vi "Wizard.vi"() -> ()   [LabVIEW 2014]
uses:
  TypeDef and Controls/QWizardMessage.ctl
  <vilib>/Utility/miscctls.llb/LVRowAndColumnUnsignedTypeDef.ctl
  Wizard Global Variable.vi
  <vilib>/Platform/browser.llb/Open URL in Default Browser (path).vi
  <vilib>/addons/_office/excel.llb/Excel Easy Table (str).vi
  <vilib>/Utility/NIReport.llb/NI_report.lvclass
  <vilib>/lvdsc/NI_DSC.lvlib
  <vilib>/addons/_office/NI_ReportGenerationToolkit.lvlib
panel:
  in  "Previous":bool
  in  "Cancel":bool
  in  "Next":bool
  in  "Tab Control":T1(tab)
  in  "Step 0 Selector":enum32{"Create", "Manage"}(radio) caption="Select an option to proceed"
  in  "what is database?":bool
  in  "Step 1 Database":enum32{"Database Ready", "Make Database"}(radio) caption="Select an option to proceed"
  out "S1 database def":string
  in  "S2 Library Name":string caption="Library Name"
  in  "S2 Database Location":path caption="Database Location"
  in  "S2 bool Library Name":enum32{"Libname:app", "Libname:user"}(radio) caption="Select an option to proceed"
  out "TextPage3":string
  in  "Bind":bool
  out "Processing 2":string
  out "S3 Status":string caption="Status"
  in  "S3 Open File Location":bool
  out "Processing":string
  in  "S4 Server IP":string="localhost" caption="Server Name/IP"
  in  "S4 Deployed Processes":i32[](listbox) caption="Deployed Processes"
  in  "S4 Remove Process":bool
  in  "S4 Get Process":bool
  in  "S4 Initialize":bool
  in  "S4 Deploy":bool
  in  "S4 SV Lib Path":path caption="Shared Variable Library Location"
  out "S5 Status":string caption="Status"
  in  "Redo":bool
  in  "Import":bool
  in  "Created Database":i32[](listbox) caption="Variables (in selected process)"
  in  "Variables":i32[](listbox) caption="Variables (in selected process)"
  in  "Deployed Pros. AP2":i32(listbox) caption="Deployed Processes"
  in  "Database Loc AP2":path caption="Database Location"
  in  "Database Name AP2":string caption="Database Name"
  # "SV Creation Wizard"
  # "This wizard assists you to create, deploy, and initialize shared variables."
  # "You have selected to create shared variables. You need to have a database."
  # "This application creates a LabVIEW library (*.lvlib) which contains shared variables. \nWhat shall be the name of the library?"
  # "The process to create shared varibles started ..."
  # "You can deploy and initialize the library.\n\nInitialization set booleans with False, strings with empty string, scalars with 0 of the same type, \n1D/2D arrays with 1D/2D arrays of size 1 with 0 or empty strings."
  # "Select a location  and a name to save the database."
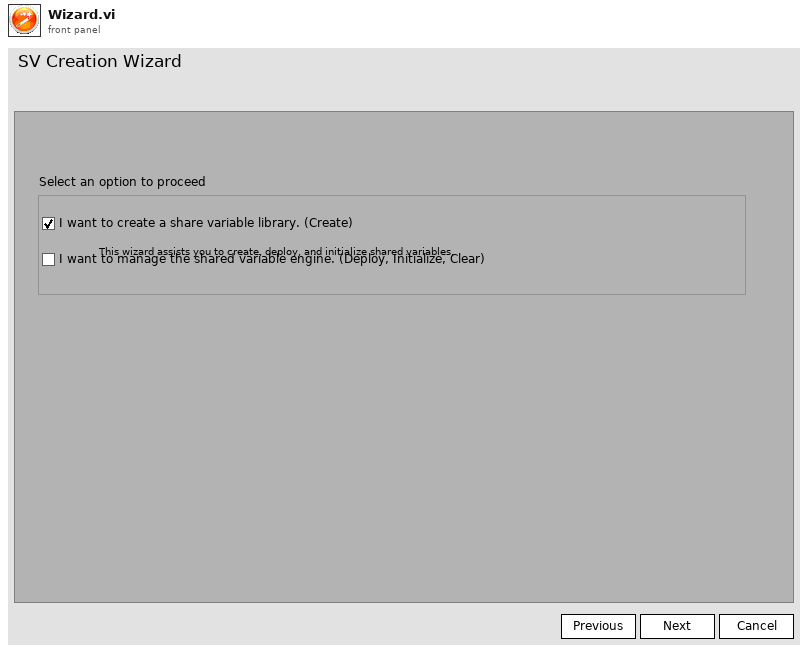
[diagram p1: front panel]
types:
  T1 = enum32{"Page 1", "Page 2", "Page 3", "Page 4", "Page 5", "Page 6", "Page 7"}
  T2 = cluster{"Number of Variables":i32, "Variable/Parent Name array":string[][], "URL array":string[], "Type array":string[]}
  T3 = typedef "QWizardMessage.ctl" = cluster{"State":enum16{"Initialize 0", "Initialize 1", "Initialize 2", "Initialize 3", "Initialize 4", "Back", "Next", "Check Database", "Get Lib Name", "Get Lib Folder", "Get Database", "Check Lib Availability", "Create SV Lib", "Check Binding", "Bind", "Get Processes", "Deploy", "Remove Process", "Clear Engine", "Initialize Process", "Get Process AP2", "Update Var AP2", "Import", "Redo", "Save Database", "Exit"}, "Data":variant}
  T4 = cluster{"Tab Pages Ref":refnum<vi>[], "Lib Name":string, "Lib Path":path, "Data":string[][], "Lib Full Path":path, "Deployed Processes":string[], "SV Info for Process":cluster{"Number of Variables":i32, "Variable/Parent Name array":string[][], "URL array":string[], "Type array":string[]}}
  T5 = typedef "LVRowAndColumnUnsignedTypeDef.ctl" = cluster{"Row":u32, "Column":u32}
  T6 = enum16{"Standard Report", "HTML", "Word", "Excel"}
  T7 = enum16{"maximized", "minimized", "normal", "no change"}
  T8 = enum16{"Initialize 0", "Initialize 1", "Initialize 2", "Initialize 3", "Initialize 4", "Back", "Next", "Check Database", "Get Lib Name", "Get Lib Folder", "Get Database", "Check Lib Availability", "Create SV Lib", "Check Binding", "Bind", "Get Processes", "Deploy", "Remove Process", "Clear Engine", "Initialize Process", "Get Process AP2", "Update Var AP2", "Import", "Redo", "Save Database", "Exit"}
  T9 = typedef "LVPoint32TypeDef.ctl" = cluster{"Horizontal":i32, "Vertical":i32}
  T10 = typedef "LVRowAndColumnTypeDef.ctl" = cluster{"Row":i32, "Column":i32}
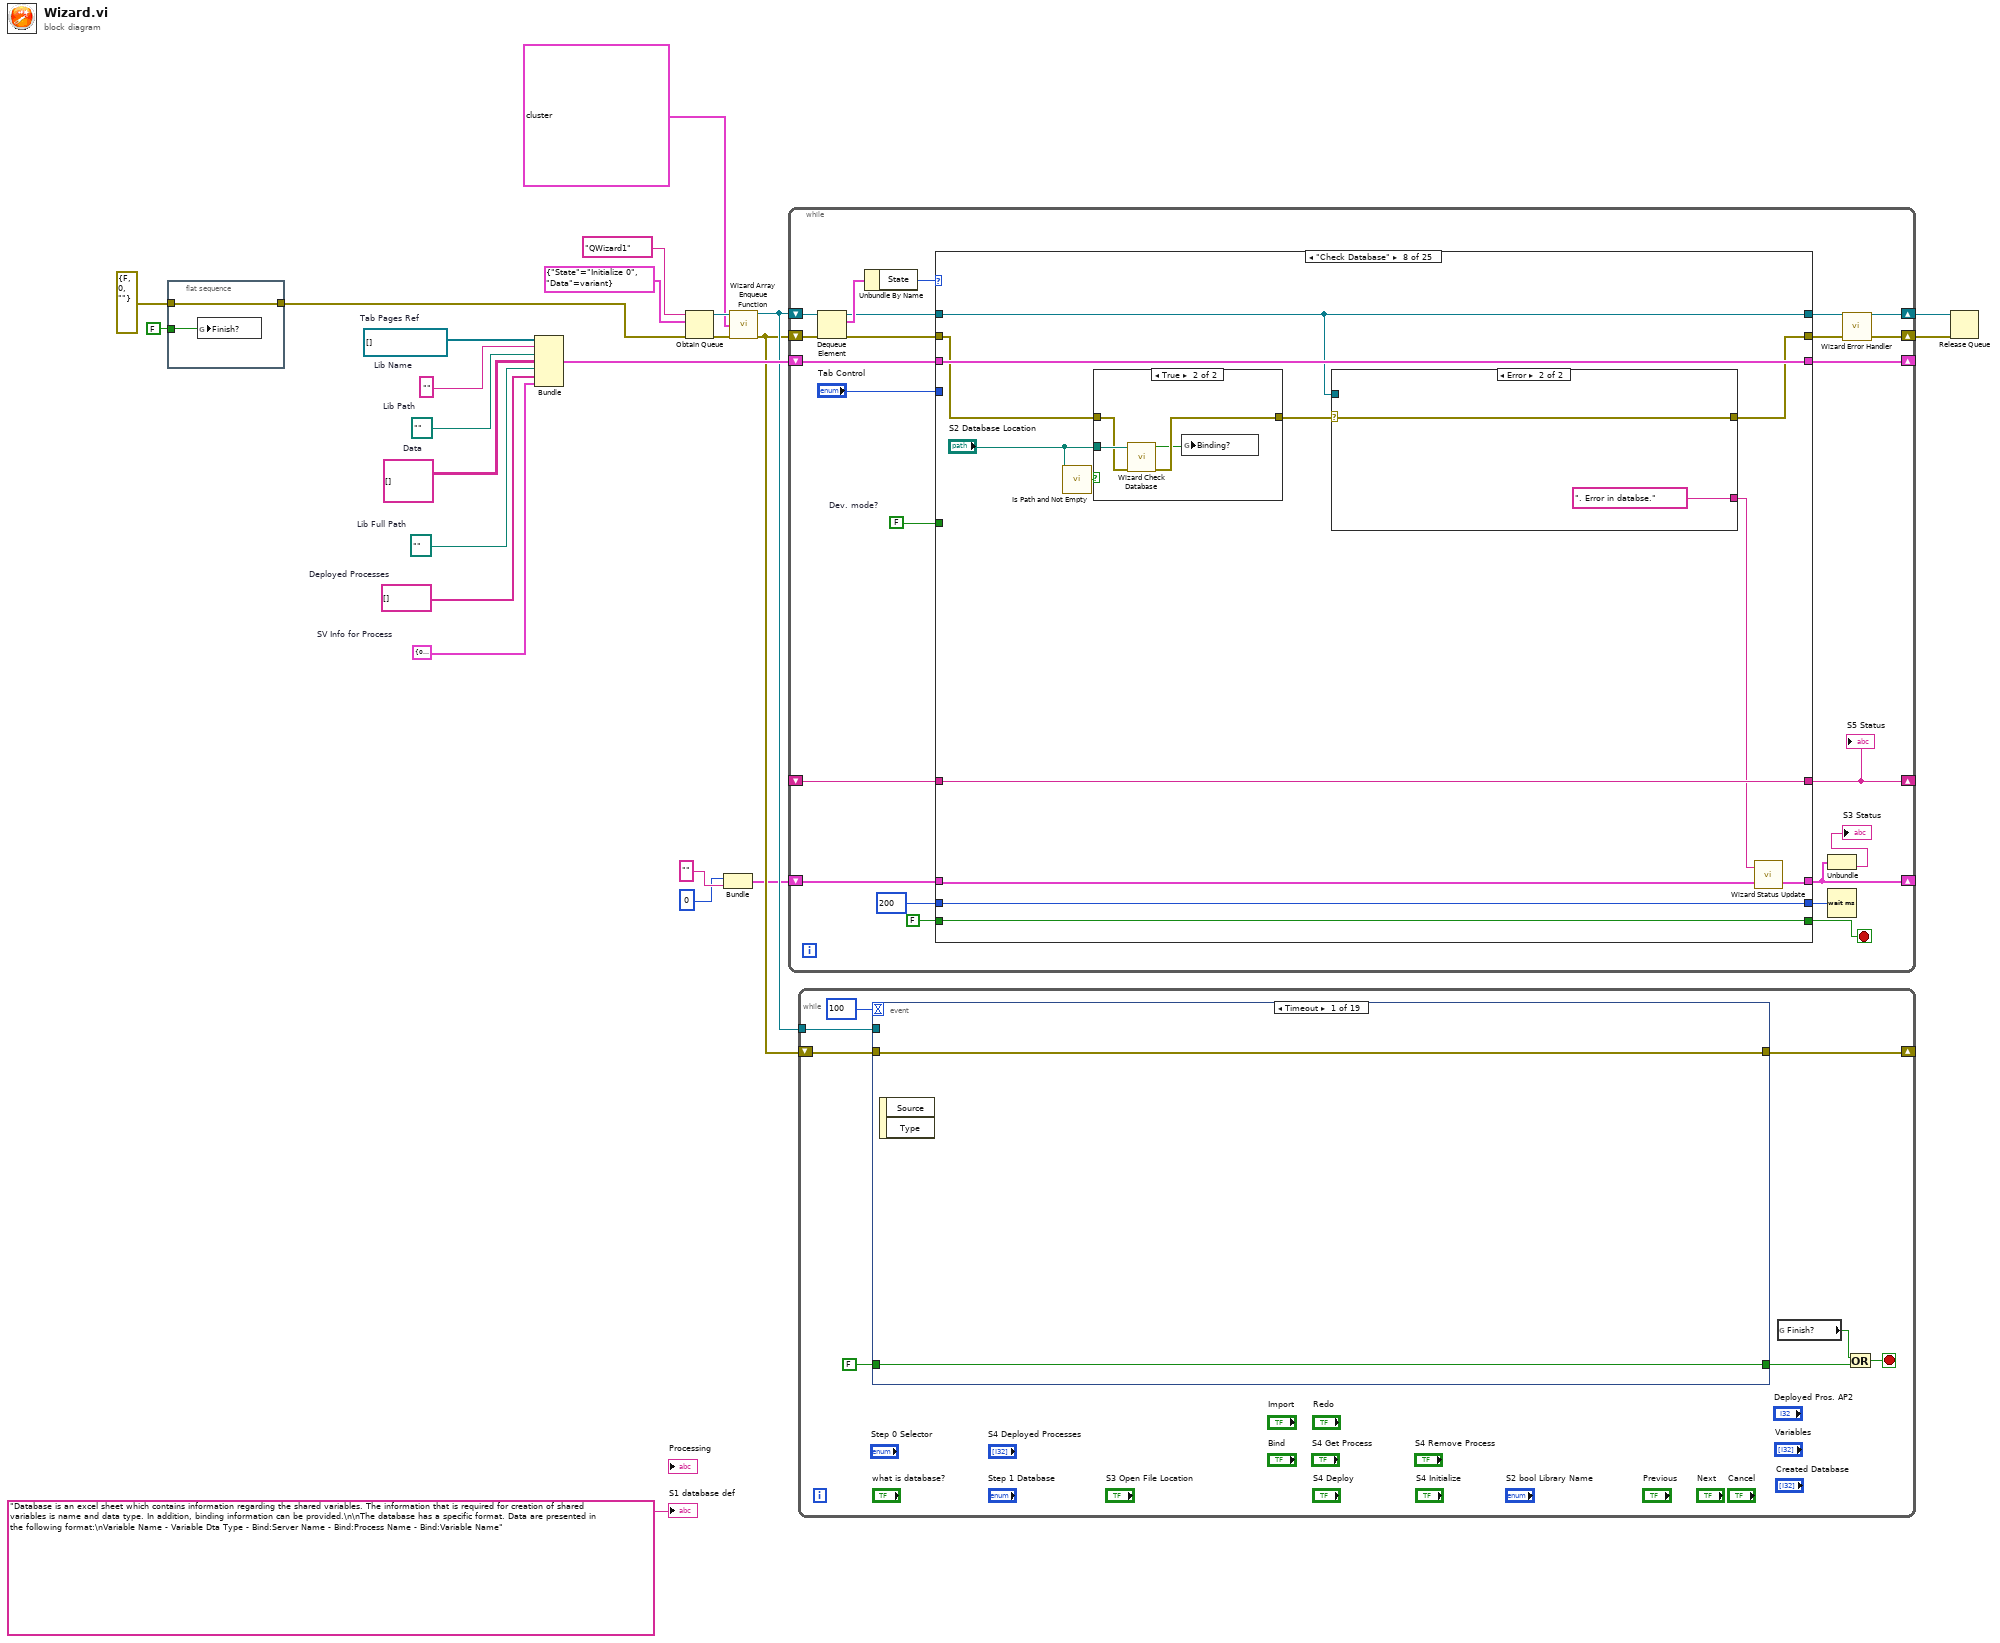
[diagram p0: block diagram]
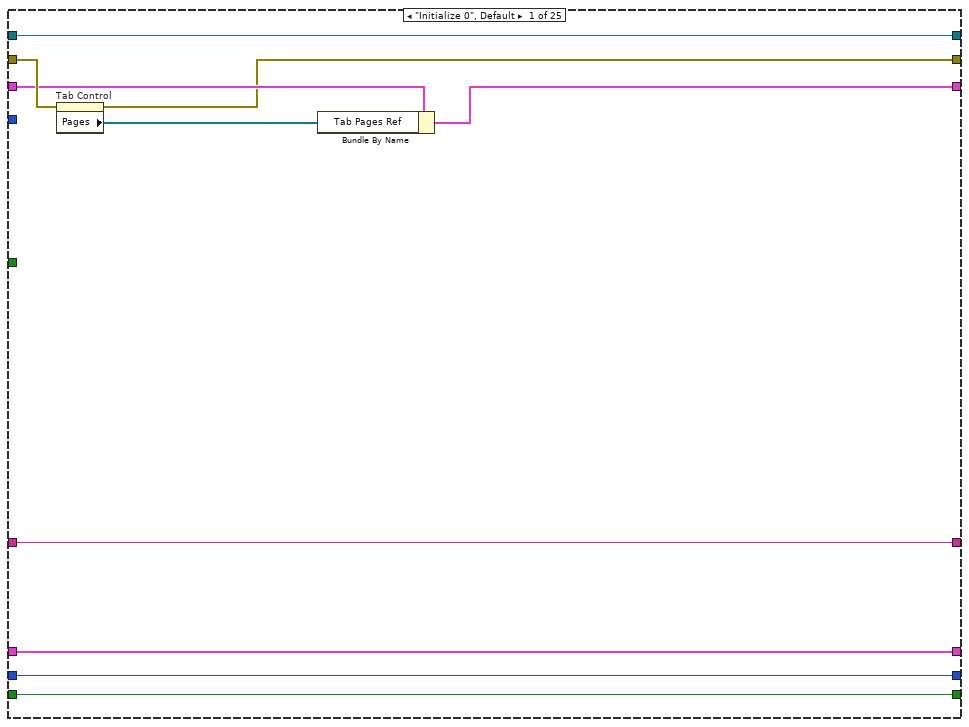
[diagram p2: hidden frame]
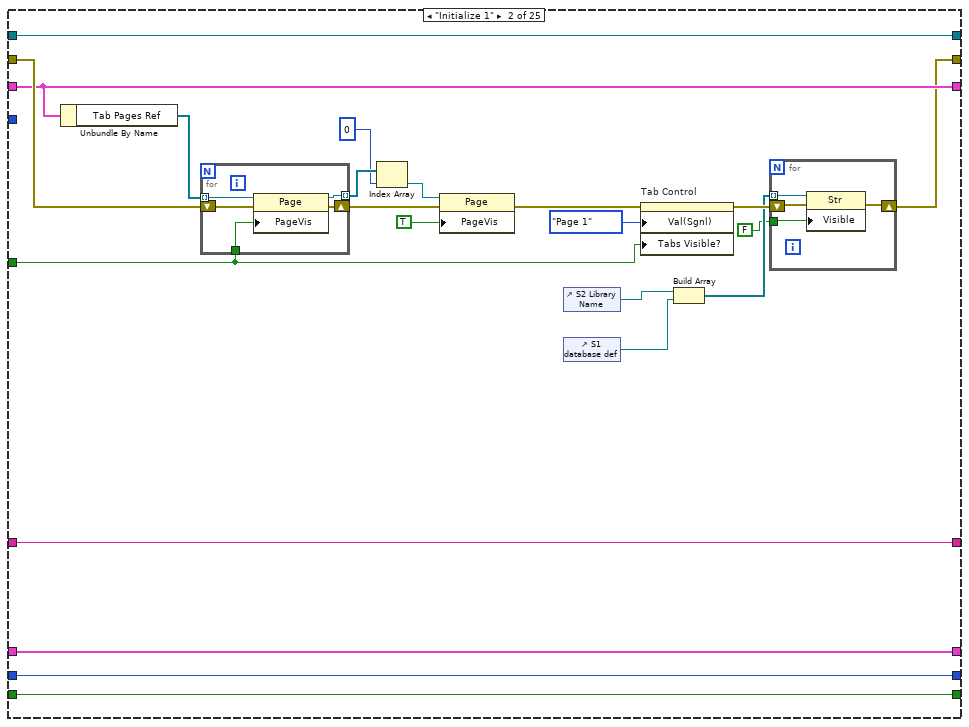
[diagram p3: hidden frame]
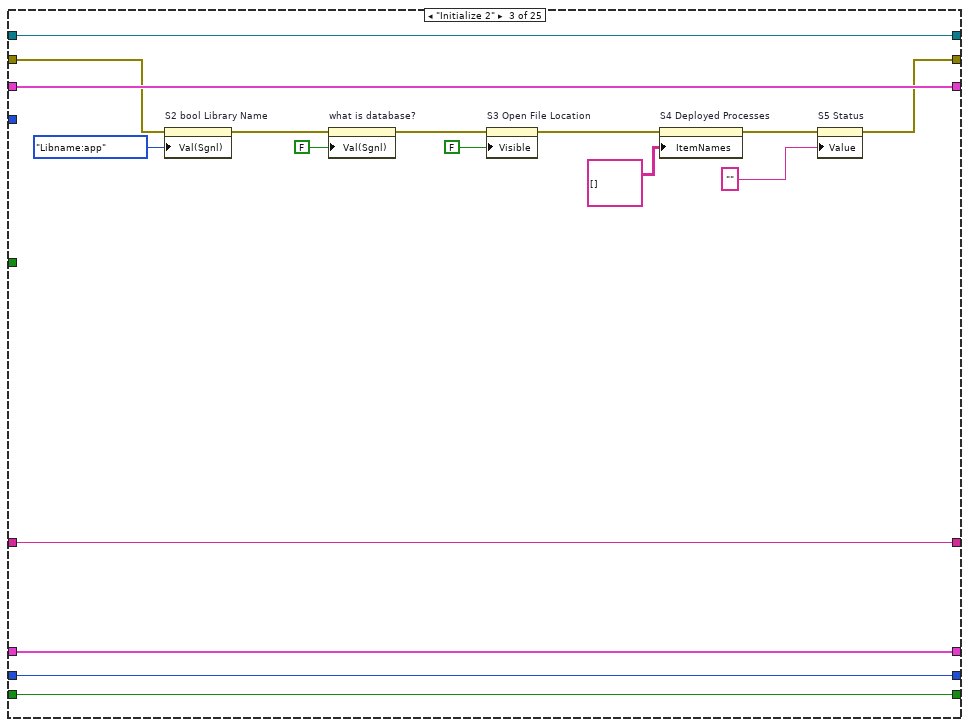
[diagram p4: hidden frame]
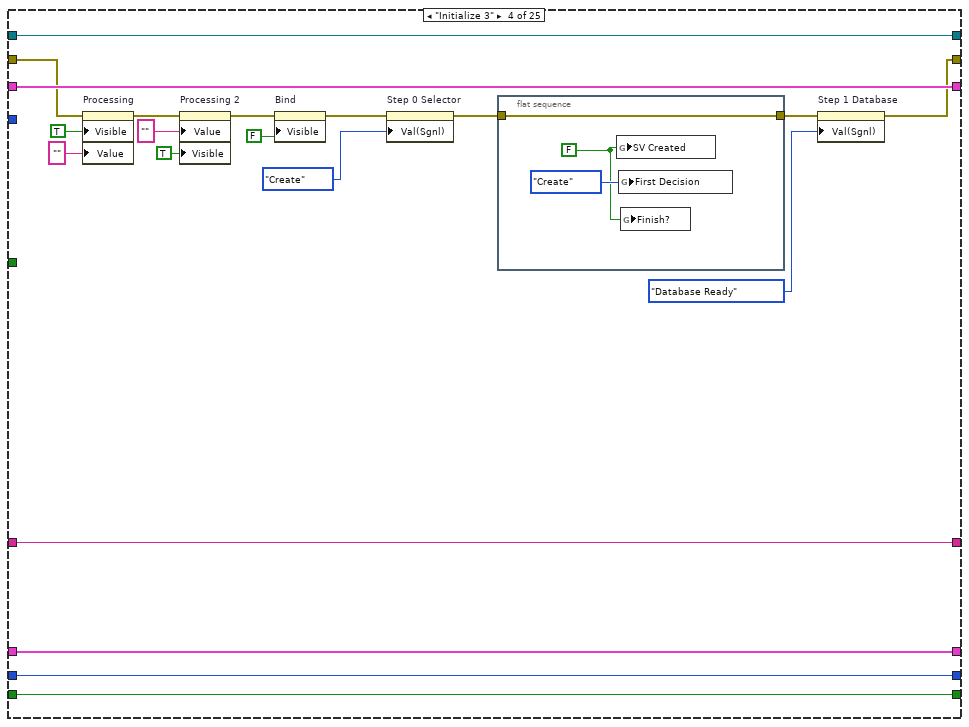
[diagram p5: hidden frame]
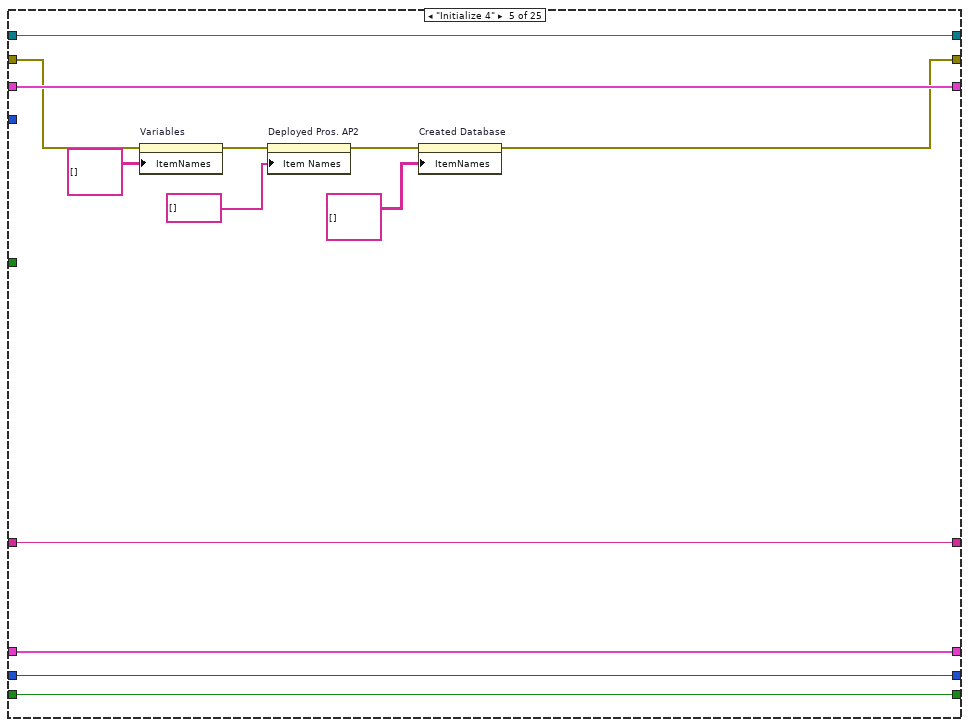
[diagram p6: hidden frame]
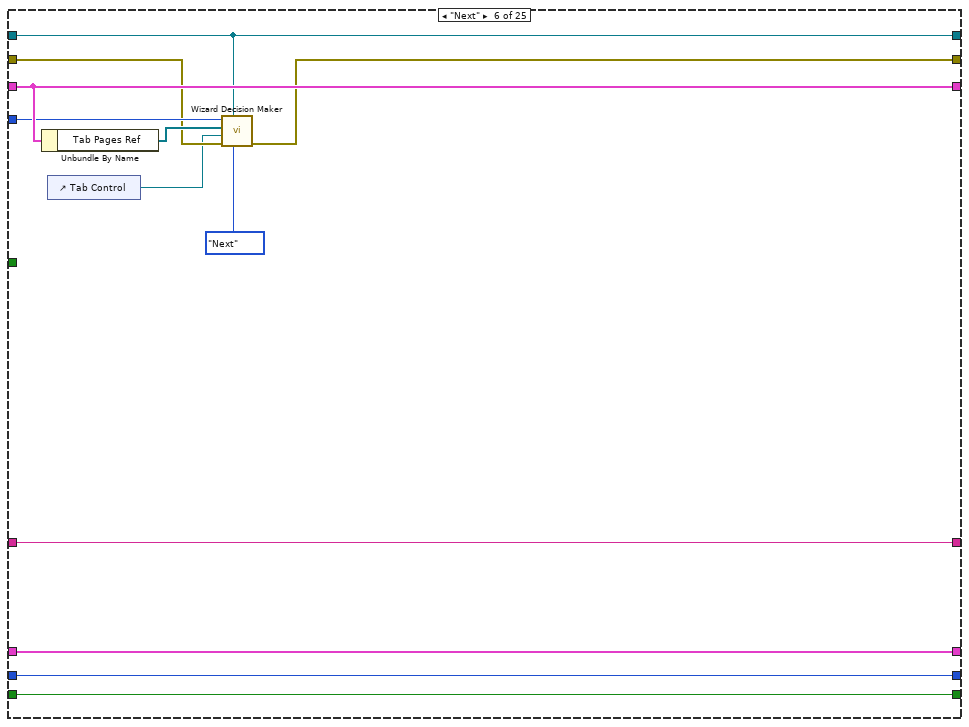
[diagram p7: hidden frame]
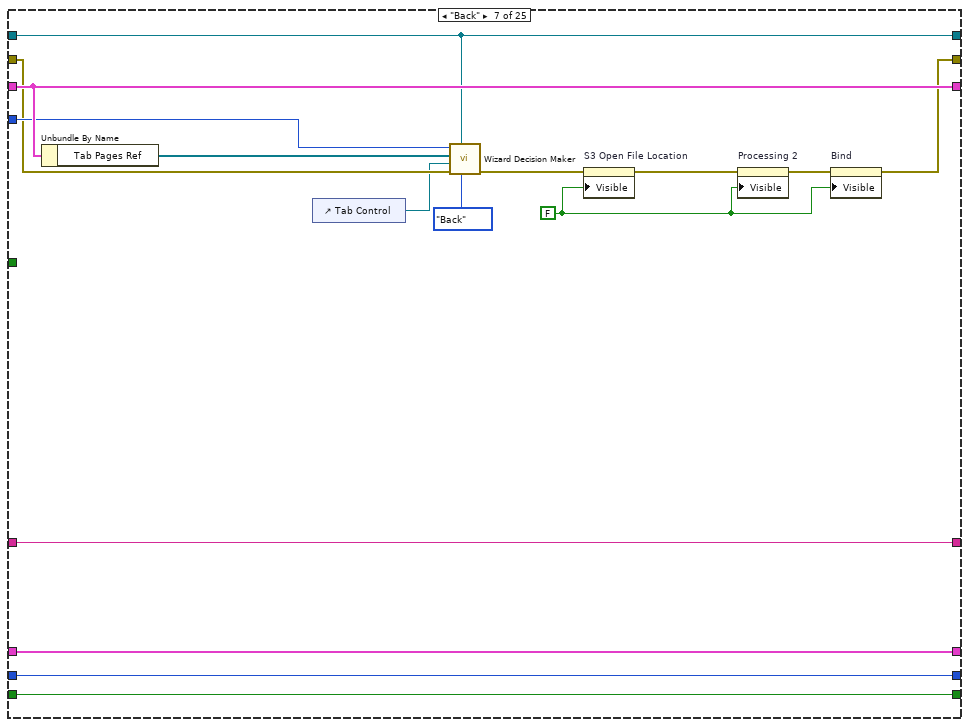
[diagram p8: hidden frame]
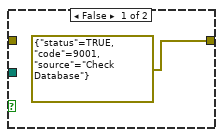
[diagram p9: hidden frame]
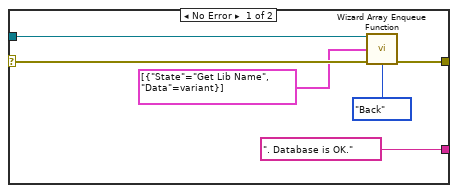
[diagram p10: hidden frame]
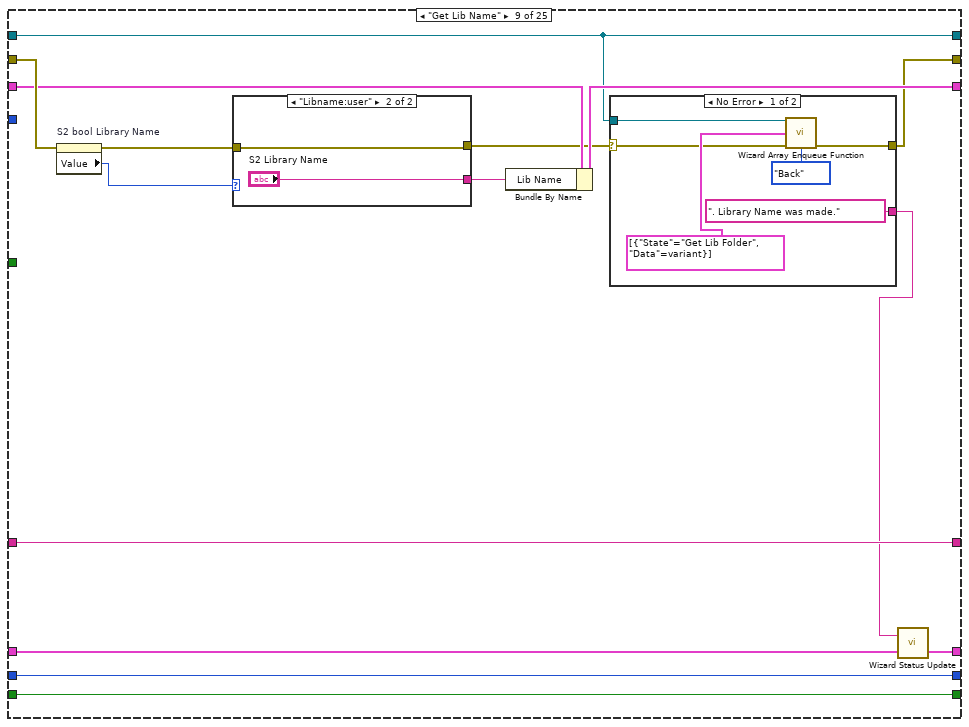
[diagram p11: hidden frame]
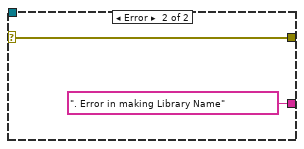
[diagram p12: hidden frame]
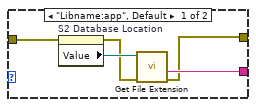
[diagram p13: hidden frame]
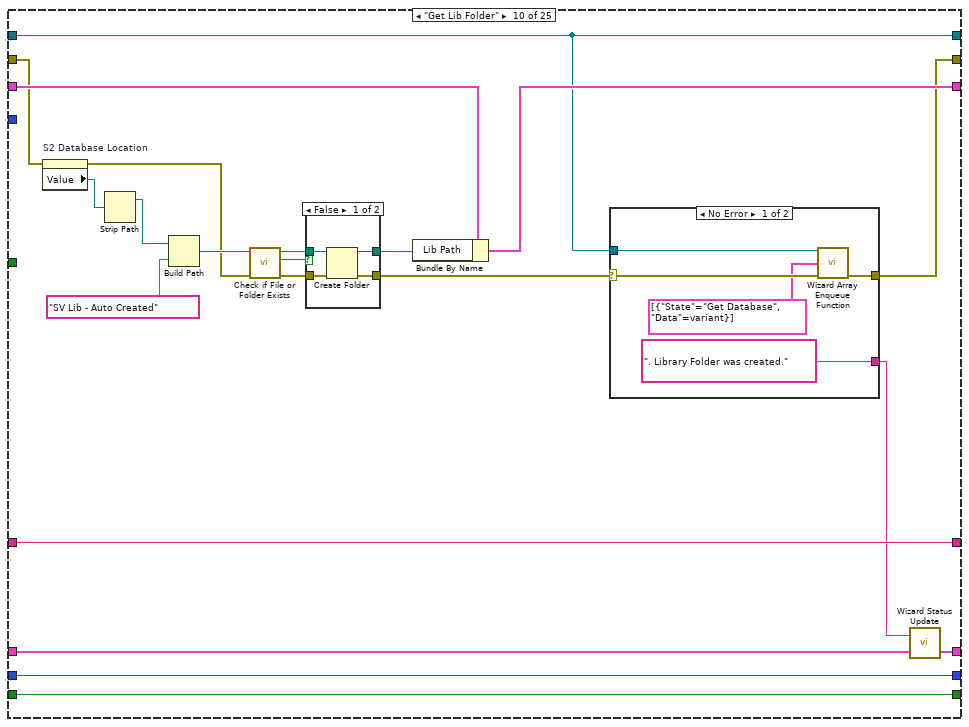
[diagram p14: hidden frame]
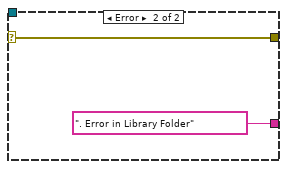
[diagram p15: hidden frame]
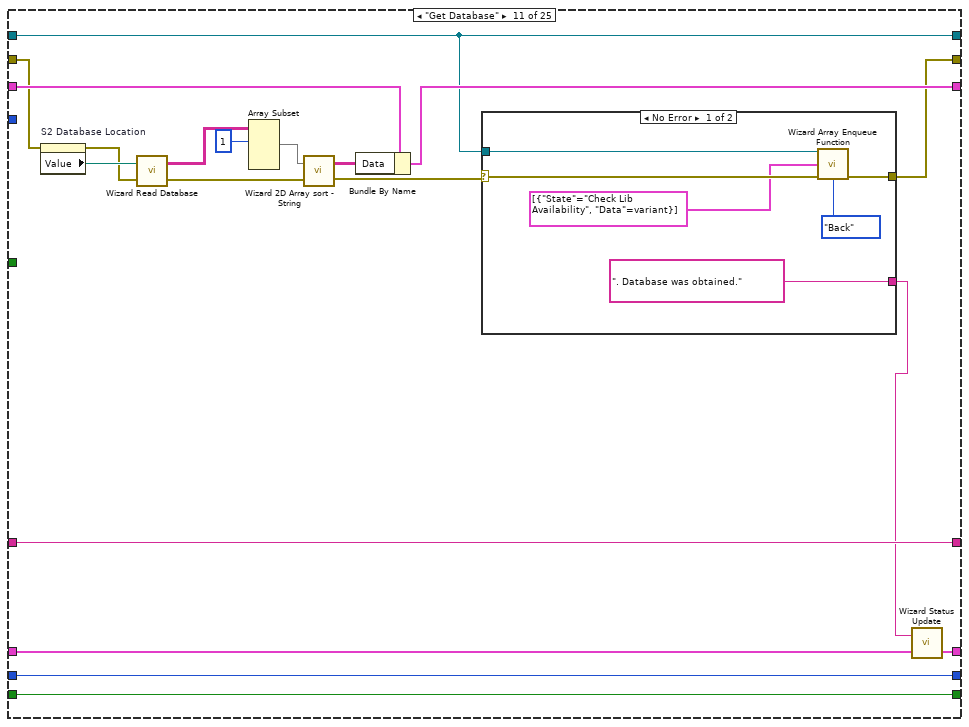
[diagram p17: hidden frame]
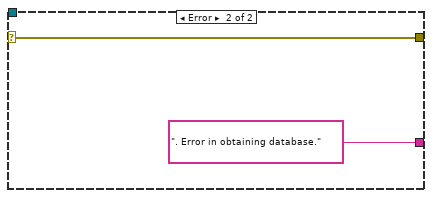
[diagram p18: hidden frame]
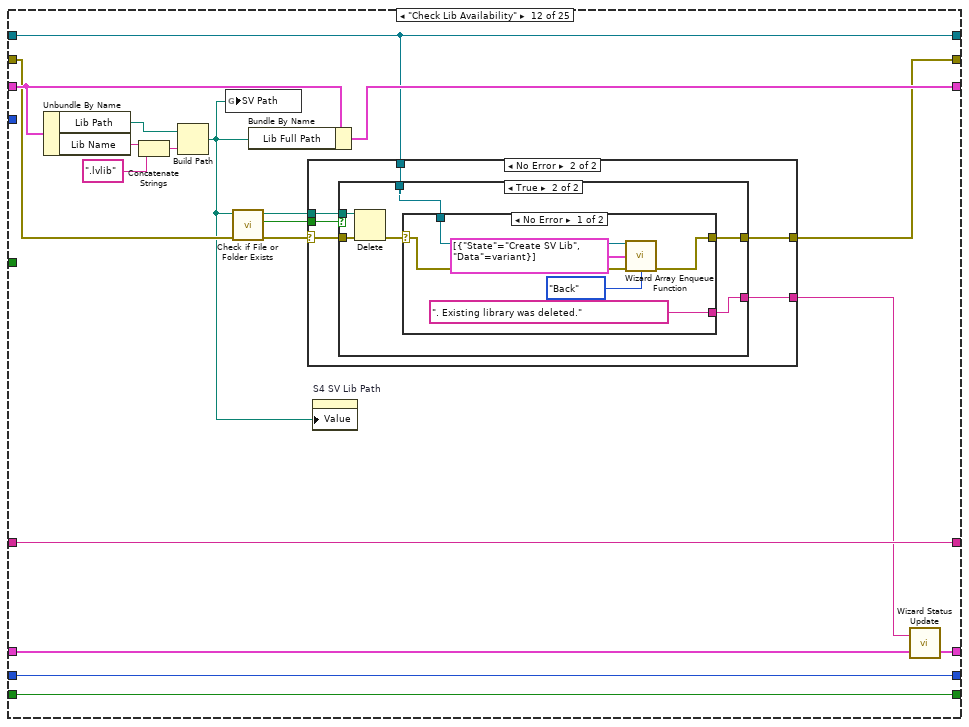
[diagram p19: hidden frame]
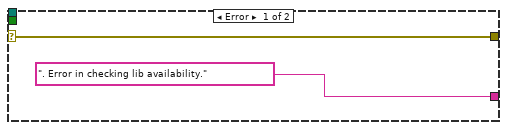
[diagram p20: hidden frame]
diagram:
  w3 = T2 {"Number of Variables"=0, "Variable/Parent Name array"=[], "URL array"=[], "Type array"=[]}  # SV Info for Process
  w7 = string[] []  # Deployed Processes
  w8 = path ""  # Lib Full Path
  w9 = string[][] []  # Data
  w10 = path ""  # Lib Path
  w11 = ""  # Lib Name
  w16 = refnum<vi>[] []  # Tab Pages Ref
  n1 = flat-sequence {
    tunnel: FALSE ("Finish?") -> [w26]
    tunnel: errorcluster {"status"=FALSE, "code"=0, "source"=""} ("error constant") -> [w25]
    tunnel: [w25] -> w4
    frame #0 {
      n2 = global write "Wizard Global Variable.vi" "Finish?"(w26) -> ()
    }
  }
  n3 = Bundle("Tab Pages Ref"=w16, "Lib Name"=w11, "Lib Path"=w10, "Data"=w9, "Lib Full Path"=w8, "Deployed Processes"=w7, "SV Info for Process"=w3) -> (w22:T4)  [unwired: 1 in]
  n4 = Obtain Queue(name (unnamed)="QWizard1", element data type=T3 {"State"=enum."Initialize 0", "Data"=variant}, error in (no error)=w4) -> (queue out=w21:refnum<queue>, error out=w20:errorcluster)  [unwired: 2 in, 1 out]
  n5 = Bundle(u32 0, "") -> (w14:cluster{u32, string})  [unwired: 1 in]
  n6 = call "Wizard Array Enqueue Function.vi"("Qref in"=w21, "Array of Messages"=T3[] [{"State"=enum."Initialize 0", "Data"=variant}, {"State"=enum."Initialize 1", "Data"=variant}, {"State"=enum."Initialize 2", "Data"=variant}, {"State"=enum."Initialize 3", "Data"=variant}, {"State"=enum."Initialize 4", "Data"=variant}], "Error in"=w20) -> ("Qref out"=w18:refnum<queue>, "Error out"=w17:errorcluster)  [unwired: 11 in]
  n7 = while {
    shift-right: [w30] -> w1
    shift-left: w17 -> [w48]
    shift-right: [w40] -> w2
    shift-left: w18 -> [w47]
    shift-right: [w41] -> _
    shift-left: w22 -> [w42]
    shift-right: [w35] -> _
    shift-left: w14 -> [w36]
    shift-right: [w28] -> _
    shift-left: _ -> [w27]
    stop <- w38 stop-if-true
    w29 = FALSE  # Dev. mode?
    n8 = Dequeue Element(queue=w47, error in (no error)=w48) -> (queue out=w45:refnum<queue>, element=w46:T3, error out=w44:errorcluster)  [unwired: 1 in, 1 out]
    n9 = Unbundle By Name(w46) -> ("State"=w43:T8)
    n10 = case shown="\"Check Database\"" w43 {
      tunnel: w45 -> [w54 w80 w105 w125 w141 w151 w166 w179 w201 w231 w267 w293 w335 w393 w413 w426 w450 w468 w497 w521 w541 w581 w619 w672 w685]
      tunnel: w44 -> [w58 w79 w103 w118 w134 w145 w163 w171 w210 w235 w266 w295 w347 w383 w407 w422 w435 w452 w487 w513 w536 w571 w606 w650 w684]
      tunnel: w42 -> [w56 w72 w106 w126 w142 w153 w169 w183 w206 w237 w274 w300 w350 w394 w409 w421 w439 w463 w498 w505 w542 w582 w620 w673 w683]
      tunnel: [w55 w72 w106 w126 w142 w153 w169 w183 w205 w236 w273 w299 w350 w394 w409 w421 w438 w463 w498 w505 w542 w582 w620 w673 w683] -> w41
      tunnel: [w54 w80 w105 w125 w141 w151 w166 w179 w201 w231 w267 w293 w335 w393 w413 w426 w450 w468 w497 w521 w541 w581 w619 w672 w685] -> w40
      tunnel: [w53 w67 w92 w108 w133 w152 w157 w180 w204 w234 w265 w294 w345 w381 w407 w419 w434 w451 w486 w506 w535 w567 w603 w646 w684] -> w31
      tunnel: FALSE -> [w52 w71 w104 w124 w140 w154 w170 w182 w211 w247 w279 w306 w354 w392 w412 w425 w449 w467 w496 w520 w540 w580 w618 w671 w686]
      tunnel: [w52 w71 w104 w124 w140 w154 w170 w182 w211 w247 w279 w306 w354 w392 w412 w425 w449 w467 w496 w520 w540 w580 w618 w671 w687] -> w38
      tunnel: "Tab Control" -> [_ _ _ _ _ w147 w165 _ _ _ _ _ _ _ _ _ _ _ _ _ _ _ _ _ _]
      tunnel: w36 -> [w51 w62 w99 w123 w139 w149 w168 w175 w198 w227 w263 w289 w337 w391 w404 w424 w448 w466 w495 w519 w539 w579 w617 w670 w682]
      tunnel: [w51 w62 w99 w123 w139 w149 w168 w176 w199 w228 w262 w290 w338 w391 w403 w424 w448 w466 w495 w519 w539 w579 w617 w670 w682] -> w35
      tunnel: u32 200 ("milliseconds to wait") -> [w50 w61 w98 w122 w138 w148 w167 w178 w203 w233 w278 w305 w353 w390 w411 w423 w447 w465 w494 w518 w538 w578 w616 w669 w681]
      tunnel: [w50 w61 w98 w122 w138 w148 w167 w178 w203 w233 w278 w305 w353 w390 w411 w423 w447 w465 w494 w518 w538 w578 w616 w669 w681] -> w32
      tunnel: w29 -> [_ w60 _ _ _ _ _ _ _ _ _ _ _ _ _ _ _ _ _ _ _ _ _ _ _]
      tunnel: [w49 w59 w91 w121 w137 w144 w160 w177 w200 w230 w264 w291 w339 w389 w410 w420 w446 w464 w493 w504 w537 w573 w610 w668 w680] -> w28
      tunnel: w27 -> [w49 w59 w91 w121 w137 w144 w160 w177 w200 w230 w264 w291 w339 w389 w410 w420 w446 w464 w493 w504 _ _ _ w668 w680]
      frame "Initialize 0", Default {
        n11 = property on="Tab Control" class="TabCtl (strict)"(error in=w58) -> (error out=w53:errorcluster, "Pages"=w57:refnum<vi>[])  [unwired: 1 in, 1 out]
        n12 = Bundle By Name(cluster=w56, "Tab Pages Ref"=w57) -> (w55:T4)
      }
      frame "Initialize 1" {
        n13 = Unbundle By Name(w72) -> ("Tab Pages Ref"=w78:refnum<vi>[])
        n14 = for {
          tunnel: w78 -> [w89] mode=indexing
          shift-right: [w87] -> w75
          shift-left: w79 -> [w88]
          tunnel: [w86] -> w77 mode=indexing
          tunnel: w60 -> [w85]
          n15 = property class="Page"(reference=w89, error in=w88, "PageVis"=w85) -> (reference out=w86:refnum<vi>, error out=w87:errorcluster)
        }
        n16 = Index Array(array=w77, index=0) -> (element=w74:refnum<vi>)
        n17 = property class="Page"(reference=w74, error in=w75, "PageVis"=TRUE ("Page Visible")) -> (error out=w70:errorcluster)  [unwired: 1 out]
        n18 = control-ref of="S2 Library Name"() -> (w66:refnum<vi>)
        n19 = control-ref of="S1 database def"() -> (w65:refnum<vi>)
        n20 = property on="Tab Control" class="TabCtl (strict)"(error in=w70, "Val(Sgnl)"=enum32{"Page 1", "Page 2", "Page 3", "Page 4"}."Page 1" ("Value (Signaling)"), "Tabs Visible?"=w60) -> (error out=w68:errorcluster)  [unwired: 1 in, 1 out]
        n21 = Build Array(w66, w65) -> (w64:refnum<vi>[])
        n22 = for {
          shift-right: [w81] -> w67
          shift-left: w68 -> [w84]
          tunnel: w64 -> [w83] mode=indexing
          tunnel: FALSE ("Visible") -> [w82]
          n23 = property class="Str"(reference=w83, error in=w84, "Visible"=w82) -> (error out=w81:errorcluster)  [unwired: 1 out]
        }
      }
      frame "Initialize 2" {
        n24 = property on="S2 bool Library Name" class="RadioBtnsControl (strict)"(error in=w103, "Val(Sgnl)"=enum32{"Libname:app", "Libname:user"}."Libname:app" ("Value (Signaling)")) -> (error out=w101:errorcluster)  [unwired: 1 in, 1 out]
        n25 = property on="what is database?" class="Bool (strict)"(error in=w101, "Val(Sgnl)"=FALSE ("Value (Signaling)")) -> (error out=w97:errorcluster)  [unwired: 1 in, 1 out]
        n26 = property on="S3 Open File Location" class="Bool"(error in=w97, "Visible"=FALSE ("Value (Signaling)")) -> (error out=w96:errorcluster)  [unwired: 1 in, 1 out]
        n27 = property on="S4 Deployed Processes" class="MCListbox (strict)"(error in=w96, "ItemNames"=string[][] [] ("Item Names")) -> (error out=w94:errorcluster)  [unwired: 1 in, 1 out]
        n28 = property on="S5 Status" class="Str"(error in=w94, "Value"="" ("S5 Status")) -> (error out=w92:errorcluster)  [unwired: 1 in, 1 out]
      }
      frame "Initialize 3" {
        n29 = property on="Processing" class="Str"(error in=w118, "Visible"=TRUE, "Value"="" ("Processing")) -> (error out=w117:errorcluster)  [unwired: 1 in, 1 out]
        n30 = property on="Processing 2" class="Str"(error in=w117, "Value"="" ("Processing 2"), "Visible"=TRUE) -> (error out=w113:errorcluster)  [unwired: 1 in, 1 out]
        n31 = property on="Bind" class="Bool"(error in=w113, "Visible"=FALSE) -> (error out=w111:errorcluster)  [unwired: 1 in, 1 out]
        n32 = property on="Step 0 Selector" class="RadioBtnsControl (strict)"(error in=w111, "Val(Sgnl)"=enum32{"Create", "Manage"}."Create" ("Value (Signaling)")) -> (error out=w110:errorcluster)  [unwired: 1 in, 1 out]
        n33 = flat-sequence {
          tunnel: w110 -> [w127]
          tunnel: [w127] -> w109
          frame #0 {
            w128 = FALSE
            n34 = global write "Wizard Global Variable.vi" "SV Created"(w128) -> ()
            n35 = global write "Wizard Global Variable.vi" "First Decision"(enum32{"Create", "Manage"}."Create" ("First Decision")) -> ()
            n36 = global write "Wizard Global Variable.vi" "Finish?"(w128) -> ()
          }
        }
        n37 = property on="Step 1 Database" class="RadioBtnsControl (strict)"(error in=w109, "Val(Sgnl)"=enum32{"Database Ready", "Make Database"}."Database Ready" ("Value (Signaling)")) -> (error out=w108:errorcluster)  [unwired: 1 in, 1 out]
      }
      frame "Initialize 4" {
        n38 = property on="Variables" class="MCListbox (strict)"(error in=w134, "ItemNames"=string[][] [] ("Item Names")) -> (error out=w136:errorcluster)  [unwired: 1 in, 1 out]
        n39 = property on="Deployed Pros. AP2" class="LstBox (strict)"(error in=w136, "Item Names"=string[] []) -> (error out=w135:errorcluster)  [unwired: 1 in, 1 out]
        n40 = property on="Created Database" class="MCListbox (strict)"(error in=w135, "ItemNames"=string[][] [] ("Item Names")) -> (error out=w133:errorcluster)  [unwired: 1 in, 1 out]
      }
      frame "Next" {
        n41 = Unbundle By Name(w153) -> ("Tab Pages Ref"=w146:refnum<vi>[])
        n42 = control-ref of="Tab Control"() -> (w143:refnum<vi>)
        n43 = call "Wizard Decision Maker.vi"("Mode"=enum16{"Next", "Back"}."Next", "Qref out"=w151, "error in"=w145, 9:"Tab Control"=w143, "Tab Pages Ref"=w146, 11:"Tab Control"=w147) -> ("error out"=w152:errorcluster)  [unwired: 5 in]
      }
      frame "Back" {
        w156 = FALSE ("Visible")
        n44 = Unbundle By Name(w169) -> ("Tab Pages Ref"=w164:refnum<vi>[])
        n45 = control-ref of="Tab Control"() -> (w155:refnum<vi>)
        n46 = call "Wizard Decision Maker.vi"("Mode"=enum16{"Next", "Back"}."Back", "Qref out"=w166, "error in"=w163, 9:"Tab Control"=w155, "Tab Pages Ref"=w164, 11:"Tab Control"=w165) -> ("error out"=w161:errorcluster)  [unwired: 5 in]
        n47 = property on="S3 Open File Location" class="Bool"(error in=w161, "Visible"=w156) -> (error out=w159:errorcluster)  [unwired: 1 in, 1 out]
        n48 = property on="Processing 2" class="Str"(error in=w159, "Visible"=w156) -> (error out=w158:errorcluster)  [unwired: 1 in, 1 out]
        n49 = property on="Bind" class="Bool"(error in=w158, "Visible"=w156) -> (error out=w157:errorcluster)  [unwired: 1 in, 1 out]
      }
      frame "Check Database" {
        n50 = call <vilib>:"Is Path and Not Empty.vi"("path"="S2 Database Location") -> ("Is Path and Not Empty?"=w172:bool)  [unwired: 4 in]
        n51 = case shown="True" w172 {
          tunnel: w171 -> [_ w187]
          tunnel: [errorcluster {"status"=TRUE, "code"=9001, "source"="Check Database"} ("error constant") w186] -> w181
          tunnel: "S2 Database Location" -> [_ w188]
          frame False {
          }
          frame True {
            n52 = call "Wizard Check Database.vi"("error in"=w187, "Database Location"=w188) -> ("error out"=w186:errorcluster, "Binding"=w185:bool)  [unwired: 8 in]
            n53 = global write "Wizard Global Variable.vi" "Binding?"(w185) -> ()
          }
        }
        n54 = case shown="Error" w181 {
          selector: w181 -> [w193 w196]
          tunnel: [w194 w196] -> w180
          tunnel: w179 -> [w192 _]
          tunnel: [". Database is OK." ("string") ". Error in databse." ("string")] -> w174
          frame No Error {
            n55 = call "Wizard Array Enqueue Function.vi"("Qref in"=w192, "Array of Messages"=T3[] [{"State"=enum."Get Lib Name", "Data"=variant}], "Error in"=w193, "Mode"=enum16{"Back", "Front", "Replace"}."Back") -> ("Error out"=w194:errorcluster)  [unwired: 10 in, 1 out]
          }
          frame Error {
          }
        }
        n56 = call "Wizard Status Update.vi"("Cluster in"=w175, "String"=w174) -> ("Cluster out"=w176:cluster{u32, string})  [unwired: 1 in]
      }
      frame "Get Lib Name" {
        n57 = property on="S2 bool Library Name" class="RadioBtnsControl (strict)"(error in=w210) -> (error out=w209:errorcluster, "Value"=w208:enum32{"Libname:app", "Libname:user"})  [unwired: 1 in, 1 out]
        n58 = case shown="\"Libname:user\"" w208 {
          tunnel: w209 -> [w224 w225]
          tunnel: [w221 "S2 Library Name"] -> w207
          tunnel: [w220 w225] -> w202
          frame "Libname:app", Default {
            n59 = property on="S2 Database Location" class="Path"(error in=w224) -> (error out=w222:errorcluster, "Value"=w223:path)  [unwired: 1 in, 1 out]
            n60 = call <vilib>:"Get File Extension.vi"("error in (no error)"=w222, "file"=w223) -> ("error out"=w220:errorcluster, "filename without extension"=w221:string)  [unwired: 6 in, 2 out]
          }
          frame "Libname:user" {
          }
        }
        n61 = Bundle By Name(cluster=w206, "Lib Name"=w207) -> (w205:T4)
        n62 = case shown="No Error" w202 {
          selector: w202 -> [w212 w219]
          tunnel: w201 -> [w216 _]
          tunnel: [w214 w219] -> w204
          tunnel: [". Library Name was made." ". Error in making Library Name"] -> w197
          frame No Error {
            n63 = call "Wizard Array Enqueue Function.vi"("Qref in"=w216, "Array of Messages"=T3[] [{"State"=enum."Get Lib Folder", "Data"=variant}], "Error in"=w212, "Mode"=enum16{"Back", "Front", "Replace"}."Back") -> ("Error out"=w214:errorcluster)  [unwired: 10 in, 1 out]
          }
          frame Error {
          }
        }
        n64 = call "Wizard Status Update.vi"("Cluster in"=w198, "String"=w197) -> ("Cluster out"=w199:cluster{u32, string})  [unwired: 1 in]
      }
      frame "Get Lib Folder" {
        n65 = property on="S2 Database Location" class="Path"(error in=w235) -> (error out=w239:errorcluster, "Value"=w246:path)  [unwired: 1 in, 1 out]
        n66 = Strip Path(path=w246) -> (stripped path=w245:path)  [unwired: 1 out]
        n67 = Build Path(base path=w245, name or relative path="SV Lib - Auto Created") -> (appended path=w243:path)
        n68 = call <vilib>:"Check if File or Folder Exists.vi"("error in (no error)"=w239, "path"=w243) -> ("error out"=w241:errorcluster, "file or folder exists?"=w240:bool, "dup path"=w242:path)  [unwired: 7 in]
        n69 = case shown="False" w240 {
          tunnel: [w258 w259] -> w238
          tunnel: [w256 w260] -> w232
          tunnel: w241 -> [w257 w260]
          tunnel: w242 -> [w255 w259]
          frame False {
            n70 = Create Folder(path (use dialog)=w255, error in=w257) -> (created path=w258:path, error out=w256:errorcluster)  [unwired: 1 in, 1 out]
          }
          frame True {
          }
        }
        n71 = Bundle By Name(cluster=w237, "Lib Path"=w238) -> (w236:T4)
        n72 = case shown="No Error" w232 {
          selector: w232 -> [w250 w254]
          tunnel: [w251 w254] -> w234
          tunnel: [". Library Folder was created." ". Error in Library Folder"] -> w229
          tunnel: w231 -> [w248 _]
          frame No Error {
            n73 = call "Wizard Array Enqueue Function.vi"("Qref in"=w248, "Array of Messages"=T3[] [{"State"=enum."Get Database", "Data"=variant}], "Error in"=w250) -> ("Error out"=w251:errorcluster)  [unwired: 11 in, 1 out]
          }
          frame Error {
          }
        }
        n74 = call "Wizard Status Update.vi"("Cluster in"=w227, "String"=w229) -> ("Cluster out"=w228:cluster{u32, string})  [unwired: 1 in]
      }
      frame "Get Database" {
        n75 = property on="S2 Database Location" class="Path"(error in=w266) -> (error out=w276:errorcluster, "Value"=w277:path)  [unwired: 1 in, 1 out]
        n76 = call "Wizard Read Database.vi"("error in (no error)"=w276, "Database Location"=w277) -> ("error out"=w272:errorcluster, "Database"=w271:string[][])
        n77 = Array Subset(array=w271, index (row)=1 ("index")) -> (w269:string[][])  [unwired: 3 in]
        n78 = call "Wizard 2D Array sort - String.vi"("error in (no error)"=w272, "Array In"=w269) -> ("error out"=w268:errorcluster, "Array Out"=w275:string[][])
        n79 = Bundle By Name(cluster=w274, "Data"=w275) -> (w273:T4)
        n80 = case shown="No Error" w268 {
          selector: w268 -> [w285 w286]
          tunnel: w267 -> [w284 _]
          tunnel: [w281 w286] -> w265
          tunnel: [". Database was obtained." ". Error in obtaining database."] -> w261
          frame No Error {
            n81 = call "Wizard Array Enqueue Function.vi"("Qref in"=w284, "Array of Messages"=T3[] [{"State"=enum."Check Lib Availability", "Data"=variant}], "Error in"=w285, "Mode"=enum16{"Back", "Front", "Replace"}."Back") -> ("Error out"=w281:errorcluster)  [unwired: 10 in, 1 out]
          }
          frame Error {
          }
        }
        n82 = call "Wizard Status Update.vi"("Cluster in"=w263, "String"=w261) -> ("Cluster out"=w262:cluster{u32, string})  [unwired: 1 in]
      }
      frame "Check Lib Availability" {
        n83 = Unbundle By Name(w300) -> ("Lib Path"=w301:path, "Lib Name"=w302:string)
        n84 = Concatenate Strings(w302, ".lvlib" ("string")) -> (w303:string)
        n85 = Build Path(base path=w301, name or relative path=w303) -> (appended path=w292:path)
        n86 = global write "Wizard Global Variable.vi" "SV Path"(w292) -> ()
        n87 = call <vilib>:"Check if File or Folder Exists.vi"("error in (no error)"=w295, "path"=w292) -> ("error out"=w298:errorcluster, "file or folder exists?"=w296:bool, "dup path"=w297:path)  [unwired: 7 in]
        n88 = Bundle By Name(cluster=w300, "Lib Full Path"=w292) -> (w299:T4)
        n89 = case shown="No Error" w298 {
          selector: w298 -> [w308 w313]
          tunnel: w297 -> [_ w311]
          tunnel: w296 -> [_ w314]
          tunnel: [w308 w312] -> w294
          tunnel: [". Error in checking lib availability." w310] -> w288
          tunnel: w293 -> [_ w309]
          frame Error {
          }
          frame No Error {
            n90 = case shown="True" w314 {
              tunnel: w313 -> [w319 w326]
              tunnel: [w318 w323] -> w312
              tunnel: w311 -> [_ w325]
              tunnel: [". Library with given name does not exist." ("string") w322] -> w310
              tunnel: w309 -> [w317 w321]
              frame False {
                n91 = call "Wizard Array Enqueue Function.vi"("Qref in"=w317, "Array of Messages"=T3[] [{"State"=enum."Create SV Lib", "Data"=variant}], "Error in"=w319, "Mode"=enum16{"Back", "Front", "Replace"}."Back") -> ("Error out"=w318:errorcluster)  [unwired: 10 in, 1 out]
              }
              frame True {
                n92 = Delete(path (use dialog)=w325, error in=w326) -> (error out=w324:errorcluster)  [unwired: 3 in, 2 out]
                n93 = case shown="No Error" w324 {
                  selector: w324 -> [w329 w334]
                  tunnel: [w331 w334] -> w323
                  tunnel: [". Existing library was deleted." ". Error in deleting existing library."] -> w322
                  tunnel: w321 -> [w330 _]
                  frame No Error {
                    n94 = call "Wizard Array Enqueue Function.vi"("Qref in"=w330, "Array of Messages"=T3[] [{"State"=enum."Create SV Lib", "Data"=variant}], "Error in"=w329, "Mode"=enum16{"Back", "Front", "Replace"}."Back") -> ("Error out"=w331:errorcluster)  [unwired: 10 in, 1 out]
                  }
                  frame Error {
                  }
                }
              }
            }
          }
        }
        n95 = property on="S4 SV Lib Path" class="Path"("Value"=w292) -> ()  [unwired: 2 in, 2 out]
        n96 = call "Wizard Status Update.vi"("Cluster in"=w289, "String"=w288) -> ("Cluster out"=w290:cluster{u32, string})  [unwired: 1 in]
      }
      frame "Create SV Lib" {
        n97 = Unbundle By Name(w350) -> ("Data"=w343:string[][], "Lib Full Path"=w342:path, "Lib Name"=w341:string)
        n98 = call <vilib>:"CreateOrAddLibraryToProject.vi"("error in (no error)"=w347) -> ("error out"=w352:errorcluster, "Library Reference Out"=w351:refnum<vi>, "Project Reference Out"=w344:refnum<vi>)  [unwired: 8 in]
        n99 = call "DatabaseToSharedVariable.vi"("error in"=w352, "database"=w343, "Library in"=w351) -> ("error out"=w348:errorcluster, "Library out"=w349:refnum<vi>)  [unwired: 6 in, 1 out]
        n100 = case shown="Error" w348 {
          selector: w348 -> [w363 w377]
          tunnel: w349 -> [w364 _]
          tunnel: [w362 ". Error in creation process."] -> w336
          tunnel: [w361 w377] -> w346
          tunnel: [w360 _] -> w340
          tunnel: w342 -> [w359 _]
          tunnel: w344 -> [w357 _]
          tunnel: w341 -> [w356 _]
          tunnel: w335 -> [w355 _]
          frame No Error {
            n101 = call "Wizard Save Library.vi"("error in (no error)"=w363, "Lib Full Path"=w359, "Library in"=w364, "Project in"=w357) -> ("error out"=w358:errorcluster)  [unwired: 7 in]
            n102 = case shown="Error" w358 {
              selector: w358 -> [w369 w375]
              tunnel: [w373 ". Error in saving shared variable library."] -> w362
              tunnel: [w367 w375] -> w361
              tunnel: [TRUE _] -> w360
              tunnel: w356 -> [w372 _]
              tunnel: w355 -> [w368 _]
              frame No Error {
                n103 = Concatenate Strings(". Shared Variable Library \"", w372, "\" was successfully created and saved.") -> (w373:string)
                n104 = call "Wizard Array Enqueue Function.vi"("Qref in"=w368, "Array of Messages"=T3[] [{"State"=enum."Check Binding", "Data"=variant}], "Error in"=w369, "Mode"=enum16{"Back", "Front", "Replace"}."Back") -> ("Error out"=w367:errorcluster)  [unwired: 10 in, 1 out]
              }
              frame Error {
              }
            }
          }
          frame Error {
          }
        }
        n105 = global write "Wizard Global Variable.vi" "SV Created"(w340) -> ()
        n106 = property on="S3 Open File Location" class="Bool"(error in=w346, "Visible"=w340) -> (error out=w345:errorcluster)  [unwired: 1 in, 1 out]
        n107 = call "Wizard Status Update.vi"("Cluster in"=w337, "String"=w336) -> ("Cluster out"=w338:cluster{u32, string})  [unwired: 1 in]
      }
      frame "Check Binding" {
        n108 = global read "Wizard Global Variable.vi" "SV Created"() -> (w387:bool)
        n109 = global read "Wizard Global Variable.vi" "Binding?"() -> (w388:bool)
        n110 = And(x=w388, y=w387) -> (x .and. y?=w386:bool)
        n111 = case shown="False" w386 {
          selector: w386 -> [w396 w399]
          tunnel: ["Although the library was created, but information for biding is not complete. Binding is not possible." "The database you selected contains binding information. Would you like to bind shared variables?"] -> w385
          tunnel: [w397 w400] -> w384
          tunnel: w383 -> [w397 w400]
          tunnel: [TRUE w399] -> w380
          tunnel: [w396 w399] -> w379
          frame False {
          }
          frame True {
          }
        }
        "Processing 2" <- w385
        n112 = property on="Processing 2" class="Str"(error in=w384, "Visible"=w380) -> (error out=w382:errorcluster)  [unwired: 1 in, 1 out]
        n113 = property on="Bind" class="Bool"(error in=w382, "Visible"=w379) -> (error out=w381:errorcluster)  [unwired: 1 in, 1 out]
      }
      frame "Bind" {
        n114 = Unbundle By Name(w409) -> ("Lib Full Path"=w406:path, "Data"=w408:string[][])
        n115 = call "BindingVI.vi"("Library Path"=w406, "error in"=w407, "Binding info"=w408) -> ("error out"=w405:errorcluster)  [unwired: 7 in, 1 out]
        n116 = case shown="No Error" w405 {
          tunnel: [". Binding was successful" ". Error while binding"] -> w402
          frame No Error {
          }
          frame Error {
          }
        }
        n117 = call "Wizard Status Update.vi"("Cluster in"=w404, "String"=w402) -> ("Cluster out"=w403:cluster{u32, string})  [unwired: 1 in]
      }
      frame "Get Process AP2" {
        n118 = call <vilib>:"Get Process List.vi"("error in (no error)"=w422) -> ("error out"=w417:errorcluster, "processes"=w418:string[])  [unwired: 9 in]
        n119 = property on="Deployed Pros. AP2" class="LstBox (strict)"(error in=w417, "Item Names"=w418, "Val(Sgnl)"=0 ("Value (Signaling)")) -> (error out=w419:errorcluster)  [unwired: 1 in, 1 out]
      }
      frame "Update Var AP2" {
        n120 = property on="Deployed Pros. AP2" class="LstBox (strict)"(error in=w435) -> (error out=w440:errorcluster, "Item Names"=w445:string[], "Value"=w444:i32)  [unwired: 1 in, 1 out]
        n121 = Index Array(array=w445, index=w444) -> (element=w443:string)
        n122 = Concatenate Strings("ni.var.psp://localhost/", w443) -> (w441:string)
        n123 = call "Get SV info.vi"("Error In"=w440, "container refnum in"=w441) -> ("Error Out"=w436:errorcluster, "Deployed Shared Variable Information"=w437:T2)  [unwired: 7 in, 1 out]
        n124 = Unbundle By Name(w437) -> ("Variable/Parent Name array"=w433:string[][])
        n125 = Bundle By Name(cluster=w439, "SV Info for Process"=w437) -> (w438:T4)
        n126 = Index Array(array=w433, index (col)=0 ("disabled index (col)")) -> (element=w431:string[])  [unwired: 1 in]
        n127 = Build Array(w431) -> (w430:string[][])
        n128 = Transpose 2D Array(2D array=w430) -> (transposed array=w429:string[][])
        n129 = property on="Variables" class="MCListbox (strict)"(error in=w436, "ItemNames"=w429, "Value"=i32[] [0] ("Variables"), "TopLeft"=T5 {"Row"=0, "Column"=0} ("Top Left Visible Cell")) -> (error out=w434:errorcluster)  [unwired: 1 in, 1 out]
      }
      frame "Import" {
        n130 = property on="Variables" class="MCListbox (strict)"(error in=w452) -> (error out=w461:errorcluster, "Value"=w462:i32[], "ItemNames"=w458:string[][])  [unwired: 1 in, 1 out]
        n131 = Unbundle By Name(w463) -> ("SV Info for Process.Variable/Parent Name array"=w460:string[][], "SV Info for Process.Type array"=w459:string[])
        n132 = for {
          tunnel: w462 -> [w479] mode=indexing
          shift-right: [w474] -> w457
          shift-left: w461 -> [w474]
          tunnel: w460 -> [w483]
          tunnel: w459 -> [w482]
          tunnel: w458 -> [w480]
          tunnel: [w475] -> w455 mode=indexing
          n133 = Index Array(array=w483, index (row)=w479) -> (element=w481:string[])  [unwired: 1 in]
          n134 = Index Array(array=w480, index (row)=w479, index (col)=1 ("disabled index (col)")) -> (element=w472:string)
          n135 = Index Array(array=w482, index=w479) -> (element=w477:string)
          n136 = Empty String/Path?(string/path=w472) -> (empty?=w473:bool)
          n137 = Index Array(array=w481) -> (element #1=w469:string, element #2=w470:string)  [unwired: 2 in]
          n138 = case shown="True" w473 {
            tunnel: w472 -> [w484 _]
            tunnel: [w484 w485] -> w471
            tunnel: w469 -> [_ w485]
            frame False {
            }
            frame True {
            }
          }
          n139 = Build Array(w471, w477, "localhost", w470, w469) -> (w475:string[])
        }
        n140 = property on="Created Database" class="MCListbox (strict)"(error in=w457) -> (error out=w454:errorcluster, "ItemNames"=w456:string[][])  [unwired: 1 in, 1 out]
        n141 = Insert Into Array(array=w456, new element=w455) -> (w453:string[][])  [unwired: 2 in]
        n142 = property on="Created Database" class="MCListbox (strict)"(error in=w454, "ItemNames"=w453) -> (error out=w451:errorcluster)  [unwired: 1 in, 1 out]
      }
      frame "Redo" {
        n143 = property on="Created Database" class="MCListbox (strict)"(error in=w487) -> (error out=w490:errorcluster, "ItemNames"=w492:string[][], "Value"=w491:i32[])  [unwired: 1 in, 1 out]
        n144 = for {
          shift-right: [w500] -> w488
          shift-left: w492 -> [w503]
          tunnel: w491 -> [w501] mode=indexing
          tunnel: w490 -> [w499]
          tunnel: [w499] -> w489
          n145 = Delete From Array(array=w503, length=1, index (row)=w501) -> (array with subset deleted=w500:string[][])  [unwired: 1 in, 1 out]
        }
        n146 = property on="Created Database" class="MCListbox (strict)"(error in=w489, "ItemNames"=w488) -> (error out=w486:errorcluster)  [unwired: 1 in, 1 out]
      }
      frame "Get Processes" {
        n147 = call <vilib>:"Get Process List.vi"("error in (no error)"=w513) -> ("error out"=w517:errorcluster, "processes"=w514:string[])  [unwired: 9 in]
        n148 = for {
          tunnel: w514 -> [w527] mode=indexing
          shift-right: [w531] -> w515
          shift-left: w517 -> [w532]
          tunnel: [w529] -> w516 mode=indexing
          tunnel: "ni.var.psp://localhost/" -> [w528]
          tunnel: [w526] -> _ mode=indexing
          n149 = Concatenate Strings(w528, w527) -> (w526:string)
          n150 = call "Get SV info.vi"("Error In"=w532, "container refnum in"=w526) -> ("Error Out"=w531:errorcluster, "Number of Variables"=w530:i32)  [unwired: 7 in, 1 out]
          n151 = Number To Decimal String(number=w530) -> (decimal integer string=w529:string)  [unwired: 1 in]
        }
        n152 = Build Array(w514, w516) -> (w511:string[][])
        n153 = Transpose 2D Array(2D array=w511) -> (transposed array=w510:string[][])
        n154 = property on="S4 Deployed Processes" class="MCListbox (strict)"(error in=w515, "ItemNames"=w510) -> (error out=w507:errorcluster)  [unwired: 1 in, 1 out]
        n155 = case shown="Error" w507 {
          selector: w507 -> [w523 w525]
          tunnel: [w523 w525] -> w506
          tunnel: "Error occured in obtaining processes from SVE." -> [_ w524]
          tunnel: [w522 w524] -> _
          tunnel: "Processes were obtained." -> [w522 _]
          frame No Error {
          }
          frame Error {
          }
        }
      }
      frame "Deploy" {
        n156 = call <vilib>:"Is Path and Not Empty.vi"("path"="S4 SV Lib Path") -> ("Is Path and Not Empty?"=w534:bool)  [unwired: 4 in]
        n157 = case shown="True" w534 {
          tunnel: ["Select a library." w554] -> w537
          tunnel: w536 -> [w544 w550]
          tunnel: [w544 w547] -> w535
          tunnel: "S4 SV Lib Path" -> [_ w545]
          frame False {
          }
          frame True {
            n158 = property on="Processing" class="Str"(error in=w550, "Visible"=FALSE) -> (error out=w551:errorcluster)  [unwired: 1 in, 1 out]
            n159 = Open Application Reference(8:w551) -> (0:w559:errorcluster, 3:w560:refnum<vi>)  [unwired: 3 in]
            n160 = invoke on="Invoke Node" class="App" method="Library.Deploy Library"(reference=w560, error in=w559, "libPath"=w545, "Dest IP Address"="S4 Server IP") -> (reference out=w556:refnum<vi>, error out=w557:errorcluster)  [unwired: 1 in, 3 out]
            n161 = Close Reference(reference=w556, error in (no error)=w557) -> (error out=w555:errorcluster)
            n162 = case shown="Error" w555 {
              selector: w555 -> [w562 _]
              tunnel: [w562 errorcluster {"status"=FALSE, "code"=0, "source"=""} ("error IO")] -> w548
              tunnel: "Deployment failed." -> [_ w564]
              tunnel: [w561 w564] -> w554
              tunnel: "Deployment was successful." -> [w561 _]
              frame No Error {
              }
              frame Error {
              }
            }
            n163 = property on="Processing" class="Str"(error in=w548, "Visible"=TRUE) -> (error out=w547:errorcluster)  [unwired: 1 in, 1 out]
          }
        }
      }
      frame "Remove Process" {
        n164 = property on="Processing" class="Str"(error in=w571, "Visible"=FALSE) -> (error out=w572:errorcluster)  [unwired: 1 in, 1 out]
        n165 = property on="S4 Deployed Processes" class="MCListbox (strict)"(error in=w572) -> (error out=w577:errorcluster, "ItemNames"=w576:string[][], "Value"=w566:i32[])  [unwired: 1 in, 1 out]
        n166 = Array Size(array=w566) -> (size(s)=w565:i32)
        n167 = Index Array(array=w576, index (col)=0 ("disabled index (col)")) -> (element=w574:string[])  [unwired: 1 in]
        n168 = case shown="1.." w565 {
          tunnel: w577 -> [w584 w592]
          tunnel: w566 -> [_ w591]
          tunnel: w574 -> [_ w590]
          tunnel: ["Select a process." w587] -> w573
          tunnel: [w584 w585] -> w569
          frame 0, Default {
          }
          frame 1.. {
            n169 = for {
              shift-right: [w597] -> w589
              shift-left: w592 -> [w598]
              tunnel: w590 -> [w601]
              tunnel: w591 -> [w600] mode=indexing
              n170 = Index Array(array=w601, index=w600) -> (element=w599:string)
              n171 = call <vilib>:"Delete Process.vi"("error in (no error)"=w598, "process name"=w599) -> ("error out"=w597:errorcluster)  [unwired: 9 in]
            }
            n172 = case shown="No Error" w589 {
              selector: w589 -> [w593 _]
              tunnel: "Process removed successfully." -> [w594 _]
              tunnel: [w594 w596] -> w587
              tunnel: "Removal failed." -> [_ w596]
              tunnel: [w593 errorcluster {"status"=FALSE, "code"=0, "source"=""} ("error IO")] -> w585
              frame No Error {
              }
              frame Error {
              }
            }
          }
        }
        n173 = property on="Processing" class="Str"(error in=w569, "Visible"=TRUE) -> (error out=w567:errorcluster)  [unwired: 1 in, 1 out]
      }
      frame "Initialize Process" {
        n174 = property on="Processing" class="Str"(error in=w606, "Visible"=FALSE) -> (error out=w607:errorcluster)  [unwired: 1 in, 1 out]
        n175 = property on="S4 Deployed Processes" class="MCListbox (strict)"(error in=w607) -> (error out=w612:errorcluster, "ItemNames"=w615:string[][], "Value"=w609:i32[])  [unwired: 1 in, 1 out]
        n176 = Array Size(array=w609) -> (size(s)=w608:i32)
        n177 = Index Array(array=w615, index (col)=0 ("disabled index (col)")) -> (element=w613:string[])  [unwired: 1 in]
        n178 = case shown="1.." w608 {
          tunnel: w613 -> [_ w631]
          tunnel: w612 -> [w622 w630]
          tunnel: "ni.var.psp://localhost/" -> [_ w629]
          tunnel: [w622 w627] -> w604
          tunnel: ["Select a process." w624] -> w610
          tunnel: w609 -> [_ w623]
          frame 0, Default {
          }
          frame 1.. {
            n179 = for {
              shift-right: [w640] -> w628
              shift-left: w630 -> [w639]
              tunnel: w631 -> [w642]
              tunnel: w623 -> [w641] mode=indexing
              tunnel: w629 -> [w637]
              n180 = Index Array(array=w642, index=w641) -> (element=w636:string)
              n181 = Concatenate Strings(w637, w636) -> (w638:string)
              n182 = call "Initialize Deployed Shared Variables.vi"("Error In"=w639, "Container refnum in"=w638) -> ("Error Out"=w640:errorcluster)  [unwired: 8 in, 1 out]
            }
            n183 = case shown="Error" w628 {
              selector: w628 -> [w633 _]
              tunnel: [w633 errorcluster {"status"=FALSE, "code"=0, "source"=""} ("error IO")] -> w627
              tunnel: "Initialization completed." -> [_ w635]
              tunnel: "Initialization completed." -> [w632 _]
              tunnel: [w632 w635] -> w624
              frame No Error {
              }
              frame Error {
              }
            }
          }
        }
        n184 = property on="Processing" class="Str"(error in=w604, "Visible"=TRUE) -> (error out=w603:errorcluster)  [unwired: 1 in, 1 out]
      }
      frame "Save Database" {
        n185 = property on="Created Database" class="MCListbox (strict)"(error in=w650) -> (error out=w651:errorcluster, "ItemNames"=w653:string[][])  [unwired: 1 in, 1 out]
        n186 = Build Array (concatenate)(string[] ["Variable Name", "Variable Data Type", "Bind:Server Name", "Bind:Process Name", "Bind:Variable Name"], w653) -> (w652:string[][])
        n187 = Concatenate Strings("Database Name AP2", ".xlsx" ("string")) -> (w660:string)
        n188 = Build Path(base path="Database Loc AP2", name or relative path=w660) -> (appended path=w645:path)
        n189 = call <vilib>:"New Report.vi"("window state (normal)"=T7."no change", "report type"=T6."Excel", "error in (no error)"=w651) -> ("report out"=w665:refnum<class "NI_report.lvclass">, "error out"=w664:errorcluster)  [unwired: 11 in]
        n190 = call-poly <vilib>:"Excel Easy Table.vi"("report in"=w665, "text data"=w652, "error in (no error)"=w664) -> ("report out"=w663:refnum<class "NI_report.lvclass">, "error out"=w662:errorcluster)  [unwired: 8 in, 3 out]
        n191 = call-dynamic "Save Report to File.vi"("report in"=w663, "report file path"=w645, "error in (no error)"=w662) -> ("report out"=w657:refnum<class "NI_report.lvclass">, "error out"=w656:errorcluster)  [unwired: 11 in]
        n192 = call-dynamic "Dispose Report.vi"("report in"=w657, "save changes? (F)"=FALSE, "error in (no error)"=w656) -> ("error out"=w649:errorcluster)  [unwired: 12 in]
        n193 = case shown="No Error" w649 {
          selector: w649 -> [w677 w678]
          tunnel: "While saving the database, an error occured." ("string") -> [_ w679]
          tunnel: "Database was saved successfully. Make sure that the following path is correct." ("string") -> [w675 _]
          tunnel: w645 -> [w676 _]
          tunnel: [w675 w679] -> w643
          tunnel: [w674 w678] -> w644
          frame No Error {
            n194 = property on="S2 Database Location" class="Path"(error in=w677, "Value"=w676) -> (error out=w674:errorcluster)  [unwired: 1 in, 1 out]
          }
          frame Error {
          }
        }
        n195 = property on="TextPage3" class="Str"(error in=w644, "Value"=w643) -> (error out=w646:errorcluster)  [unwired: 1 in, 1 out]
      }
      frame "Exit" {
        n196 = Not(x=w686) -> (.not. x?=w687:bool)
      }
    }
    "S5 Status" <- w28
    n197 = Unbundle(w35) -> (→"S3 Status":string)  [unwired: 1 out]
    n198 = Wait (ms)(milliseconds to wait=w32) -> ()  [unwired: 1 out]
    n199 = call "Wizard Error Handler.vi"("error in"=w31) -> ("error out"=w30:errorcluster)  [unwired: 4 in]
  }
  n200 = while {
    tunnel: w18 -> [w695]
    shift-right: [w693] -> _
    shift-left: w17 -> [w694]
    stop <- w690 stop-if-true
    n201 = event shown="[0] Timeout" {
      selector: _ -> [_ _ _ _ _ _ _ _ _ _ _ _ _ _ _ _ _ _ _]
      dyn-events: _ -> [_ _ _ _ _ _ _ _ _ _ _ _ _ _ _ _ _ _ _]
      timeout: 100 -> [_ _ _ _ _ _ _ _ _ _ _ _ _ _ _ _ _ _ _]
      tunnel: w695 -> [_ w704 w709 w715 _ _ w727 w733 w739 w745 w751 _ _ _ _ w798 _ w809 w829]
      tunnel: w694 -> [w696 w703 w708 w714 w717 w721 w726 w732 w738 w744 w750 w755 w760 w767 w771 w797 w804 w813 w833]
      tunnel: [w696 w702 w705 w711 w717 w721 w725 w729 w735 w741 w747 w754 w759 w766 w773 w796 w800 w807 w827] -> w693
      tunnel: FALSE -> [w697 w698 w710 w716 w719 w722 w728 w734 w740 w746 w752 w756 w761 w768 w780 w799 w805 w814 w834]
      tunnel: [w697 w699 w710 w716 w719 w722 w728 w734 w740 w746 w752 w756 w761 w768 w780 w799 w805 w814 w834] -> w689
      event Timeout {
        n202 = event-data() -> ()  [unwired: 1 in, 2 out]
      }
      event "Cancel": Value Change {
        n203 = event-data() -> ()  [unwired: 1 in, 6 out]
        n204 = call "Wizard Array Enqueue Function.vi"("Qref in"=w704, "Array of Messages"=T3[] [{"State"=enum."Exit", "Data"=variant}], "Error in"=w703, "Mode"=enum16{"Back", "Front", "Replace"}."Replace") -> ("Error out"=w702:errorcluster)  [unwired: 10 in, 1 out]
        n205 = Not(x=w698) -> (.not. x?=w699:bool)
      }
      event "Next": Value Change {
        n206 = event-data() -> ()  [unwired: 1 in, 6 out]
        n207 = call "Wizard Array Enqueue Function.vi"("Qref in"=w709, "Array of Messages"=T3[] [{"State"=enum."Next", "Data"=variant}], "Error in"=w708, "Mode"=enum16{"Back", "Front", "Replace"}."Back") -> ("Error out"=w705:errorcluster)  [unwired: 10 in, 1 out]
      }
      event "Previous": Value Change {
        n208 = event-data() -> ()  [unwired: 1 in, 6 out]
        n209 = call "Wizard Array Enqueue Function.vi"("Qref in"=w715, "Array of Messages"=T3[] [{"State"=enum."Back", "Data"=variant}], "Error in"=w714, "Mode"=enum16{"Back", "Front", "Replace"}."Back") -> ("Error out"=w711:errorcluster)  [unwired: 10 in, 1 out]
      }
      event "Step 0 Selector": Value Change {
        n210 = event-data() -> ("NewVal"=w718:enum32{"Create", "Manage"})  [unwired: 1 in]
        n211 = global write "Wizard Global Variable.vi" "First Decision"(w718) -> ()
      }
      event "Step 1 Database": Value Change {
        n212 = event-data() -> ("NewVal"=w720:enum32{"Database Ready", "Make Database"})  [unwired: 1 in]
        n213 = global write "Wizard Global Variable.vi" "Second Decision"(w720) -> ()
      }
      event "Bind": Value Change {
        n214 = event-data() -> ()  [unwired: 1 in, 6 out]
        n215 = call "Wizard Array Enqueue Function.vi"("Qref in"=w727, "Array of Messages"=T3[] [{"State"=enum."Bind", "Data"=variant}], "Error in"=w726, "Mode"=enum16{"Back", "Front", "Replace"}."Back") -> ("Error out"=w725:errorcluster)  [unwired: 10 in, 1 out]
      }
      event "S4 Get Process": Value Change {
        n216 = event-data() -> ()  [unwired: 1 in, 6 out]
        n217 = call "Wizard Array Enqueue Function.vi"("Qref in"=w733, "Array of Messages"=T3[] [{"State"=enum."Get Processes", "Data"=variant}], "Error in"=w732, "Mode"=enum16{"Back", "Front", "Replace"}."Back") -> ("Error out"=w729:errorcluster)  [unwired: 10 in, 1 out]
      }
      event "S4 Deploy": Value Change {
        n218 = event-data() -> ()  [unwired: 1 in, 6 out]
        n219 = call "Wizard Array Enqueue Function.vi"("Qref in"=w739, "Array of Messages"=T3[] [{"State"=enum."Deploy", "Data"=variant}, {"State"=enum."Get Processes", "Data"=variant}], "Error in"=w738, "Mode"=enum16{"Back", "Front", "Replace"}."Back") -> ("Error out"=w735:errorcluster)  [unwired: 10 in, 1 out]
      }
      event "S4 Remove Process": Value Change {
        n220 = event-data() -> ()  [unwired: 1 in, 6 out]
        n221 = call "Wizard Array Enqueue Function.vi"("Qref in"=w745, "Array of Messages"=T3[] [{"State"=enum."Remove Process", "Data"=variant}, {"State"=enum."Get Processes", "Data"=variant}], "Error in"=w744, "Mode"=enum16{"Back", "Front", "Replace"}."Back") -> ("Error out"=w741:errorcluster)  [unwired: 10 in, 1 out]
      }
      event "S4 Initialize": Value Change {
        n222 = event-data() -> ()  [unwired: 1 in, 6 out]
        n223 = call "Wizard Array Enqueue Function.vi"("Qref in"=w751, "Array of Messages"=T3[] [{"State"=enum."Initialize Process", "Data"=variant}, {"State"=enum."Get Processes", "Data"=variant}], "Error in"=w750, "Mode"=enum16{"Back", "Front", "Replace"}."Back") -> ("Error out"=w747:errorcluster)  [unwired: 10 in, 1 out]
      }
      event "what is database?": Value Change {
        n224 = event-data() -> ("NewVal"=w753:bool)  [unwired: 1 in, 5 out]
        n225 = property on="S1 database def" class="Str"(error in=w755, "Visible"=w753) -> (error out=w754:errorcluster)  [unwired: 1 in, 1 out]
      }
      event "S2 bool Library Name": Value Change {
        n226 = event-data() -> ("NewVal"=w758:enum32{"Libname:app", "Libname:user"})  [unwired: 1 in]
        n227 = case shown="\"Libname:user\"" w758 {
          tunnel: [FALSE ("Visible") TRUE ("Visible")] -> w757
          frame "Libname:app", Default {
          }
          frame "Libname:user" {
          }
        }
        n228 = property on="S2 Library Name" class="Str"(error in=w760, "Visible"=w757) -> (error out=w759:errorcluster)  [unwired: 1 in, 1 out]
      }
      event "S3 Open File Location": Value Change {
        n229 = event-data() -> ()  [unwired: 1 in, 6 out]
        n230 = global read "Wizard Global Variable.vi" "SV Path"() -> (w765:path)
        n231 = Strip Path(path=w765) -> (stripped path=w764:path)  [unwired: 1 out]
        n232 = call-poly <vilib>:"Open URL in Default Browser.vi"("error in (no error)"=w767, "path"=w764) -> ("error out"=w766:errorcluster)  [unwired: 4 in, 1 out]
      }
      event "Tab Control": Value Change {
        n233 = event-data() -> ("NewVal"=w779:T1)  [unwired: 1 in, 5 out]
        n234 = control-ref of="Previous"() -> (w778:refnum<vi>)
        n235 = control-ref of="Next"() -> (w777:refnum<vi>)
        n236 = property on="Step 1 Database" class="RadioBtnsControl (strict)"(error in=w771) -> (error out=w770:errorcluster, "Value"=w769:enum32{"Database Ready", "Make Database"})  [unwired: 1 in, 1 out]
        n237 = case shown="\"Page 4\"" w779 {
          tunnel: w778 -> [_ _ _ _ _]
          tunnel: w777 -> [w781 w783 w787 w791 w794]
          tunnel: [w781 w783 w787 w791 w794] -> w776
          tunnel: [w782 w784 w788 w792 "Finish"] -> w775
          tunnel: "Next" -> [w782 w784 w788 w792 _]
          tunnel: [_ _ w786 _ _] -> w772
          tunnel: w769 -> [_ _ w785 _ _]
          frame "Page 1", Default {
          }
          frame "Page 2" {
          }
          frame "Page 3" {
            n238 = case shown="\"Make Database\"" w785 {
              tunnel: ["You have already prepared the databse. Please locate the database." "Database was saved successfully. Make sure that the following path is correct."] -> w786
              frame "Database Ready", Default {
              }
              frame "Make Database" {
              }
            }
          }
          frame "Page 4" {
          }
          frame "Page 5" {
          }
        }
        "TextPage3" <- w772
        n239 = property class="Bool"(reference=w776, error in=w770, "BoolText.Text"=w775) -> (error out=w773:errorcluster)  [unwired: 1 out]
      }
      event "Deployed Pros. AP2": Value Change {
        n240 = event-data() -> ()  [unwired: 1 in, 6 out]
        n241 = call "Wizard Array Enqueue Function.vi"("Qref in"=w798, "Array of Messages"=T3[] [{"State"=enum."Update Var AP2", "Data"=variant}], "Error in"=w797) -> ("Error out"=w796:errorcluster)  [unwired: 11 in, 1 out]
      }
      event "Variables": Mouse Down {
        n242 = event-data() -> ("Coords"=w803:T9)  [unwired: 1 in, 1 out]
        n243 = invoke on="Variables" class="MCListbox (strict)" method="Point To Row Column"(error in=w804, "Point"=w803) -> (error out=w802:errorcluster, "CellPosition"=w801:T10)  [unwired: 5 in, 5 out]
        n244 = property on="Variables" class="MCListbox (strict)"(error in=w802, "EditPos"=w801) -> (error out=w800:errorcluster)  [unwired: 1 in, 1 out]
      }
      event "Import": Value Change {
        n245 = event-data() -> ()  [unwired: 1 in, 6 out]
        n246 = property on="Variables" class="MCListbox (strict)"(error in=w813) -> (error out=w808:errorcluster, "Value"=w812:i32[])  [unwired: 1 in, 1 out]
        n247 = Array Size(array=w812) -> (size(s)=w811:i32)
        n248 = Greater Than 0?(x=w811) -> (x > 0?=w810:bool)
        n249 = case shown="True" w810 {
          tunnel: w809 -> [_ w825]
          tunnel: w808 -> [w816 w824]
          tunnel: [w816 w821] -> w807
          tunnel: [0 w817] -> w806
          frame False {
          }
          frame True {
            n250 = call "Wizard Array Enqueue Function.vi"("Qref in"=w825, "Array of Messages"=T3[] [{"State"=enum."Import", "Data"=variant}], "Error in"=w824) -> ("Error out"=w822:errorcluster)  [unwired: 11 in, 1 out]
            n251 = property on="Created Database" class="MCListbox (strict)"(error in=w822) -> (error out=w821:errorcluster, "ItemNames"=w820:string[][])  [unwired: 1 in, 1 out]
            n252 = Array Size(array=w820) -> (size(s)=w819:i32[])
            n253 = Index Array(array=w819, index=0) -> (element=w817:i32)
          }
        }
        n254 = global write "Wizard Global Variable.vi" "no. Imported Var"(w806) -> ()
      }
      event "Redo": Value Change {
        n255 = event-data() -> ()  [unwired: 1 in, 6 out]
        n256 = property on="Created Database" class="MCListbox (strict)"(error in=w833) -> (error out=w828:errorcluster, "Value"=w832:i32[])  [unwired: 1 in, 1 out]
        n257 = Array Size(array=w832) -> (size(s)=w831:i32)
        n258 = Greater Than 0?(x=w831) -> (x > 0?=w830:bool)
        n259 = case shown="True" w830 {
          tunnel: w829 -> [_ w845]
          tunnel: w828 -> [w836 w844]
          tunnel: [w836 w841] -> w827
          tunnel: [0 w837] -> w826
          frame False {
          }
          frame True {
            n260 = call "Wizard Array Enqueue Function.vi"("Qref in"=w845, "Array of Messages"=T3[] [{"State"=enum."Redo", "Data"=variant}], "Error in"=w844) -> ("Error out"=w842:errorcluster)  [unwired: 11 in, 1 out]
            n261 = property on="Created Database" class="MCListbox (strict)"(error in=w842) -> (error out=w841:errorcluster, "ItemNames"=w840:string[][])  [unwired: 1 in, 1 out]
            n262 = Array Size(array=w840) -> (size(s)=w839:i32[])
            n263 = Index Array(array=w839, index=0) -> (element=w837:i32)
          }
        }
        n264 = global write "Wizard Global Variable.vi" "no. Imported Var"(w826) -> ()
      }
    }
    n265 = global read "Wizard Global Variable.vi" "Finish?"() -> (w691:bool)
    n266 = Or(x=w691, y=w689) -> (x .or. y?=w690:bool)
  }
  n267 = Release Queue(queue=w2, error in (no error)=w1) -> ()  [unwired: 1 in, 3 out]
  "S1 database def" <- "Database is an excel sheet which contains information regarding the shared variables. The information that is required for creation of shared variables is name and data type. In addition, binding information can be provided.\n\nThe database has a specific format. Data are presented in the following format:\nVariable Name - Variable Dta Type - Bind:Server Name - Bind:Process Name - Bind:Variable Name" ("S1 database def")
